vi "FPGA Sensing.vi"(8 "Error In":errorcluster, 11 "FPGA VI Reference In":refnum<k20>) -> (0 "Error Out":errorcluster, 2 "SSG Data Out":T1 {"SSG Active Current" format="%2.1f"; "PV Reactive Power (L1)" format="%2.1f"; "PV Reactive Power (L2)" format="%2.1f"; "PV Total Reactive Power" format="%2.1f"; "Gen Reactive Power (L1)" format="%2.1f"; "Gen Reactive Power (L2)" format="%2.1f"; "Gen Total Reactive Power" format="%2.1f"; "SSG Reactive Power (L1)" format="%2.1f"; "SSG Reactive Power (L2)" format="%2.1f"; "SSG Total Reactive Power" format="%2.1f"; "PV Total Current" format="%2.1f"; "PV Total Voltage" format="%2.1f"; "PV Active Power (L1)" format="%2.1f"; "PV Active Power (L2)" format="%2.1f"; "PV App Power (L1)" format="%2.1f"; "PV App Power (L2)" format="%2.1f"; "PV Total Active Power" format="%2.1f"; "PV Total App Power" format="%2.1f"; "PV Arms (L1)" format="%2.1f"; "PV Arms (L2)" format="%2.1f"; "PV Vrms (L1)" format="%2.1f"; "PV Vrms (L2)" format="%2.1f"; "Gen Total Current" format="%2.1f"; "SSG Total Current" format="%2.1f"; "Gen Total Voltage" format="%2.1f"; "SSG Total Voltage" format="%2.1f"; "Gen Active Power (L1)" format="%2.1f"; "Gen Active Power (L2)" format="%2.1f"; "SSG Active Power (L1)" format="%2.1f"; "SSG Active Power (L2)" format="%2.1f"; "Gen App Power (L1)" format="%2.1f"; "Gen App Power (L2)" format="%2.1f"; "SSG App Power (L1)" format="%2.1f"; "SSG App Power (L2)" format="%2.1f"; "Gen Total Active Power" format="%2.1f"; "Gen Total App Power" format="%2.1f"; "Gen Arms (L1)" format="%2.1f"; "Gen Arms (L2)" format="%2.1f"; "Gen Vrms (L1)" format="%2.1f"; "Gen Vrms (L2)" format="%2.1f"; "SSG Total Active Power" format="%2.1f"; "SSG Total App Power" format="%2.1f"; "SSG Arms (L1)" format="%2.1f"; "SSG Arms (L2)" format="%2.1f"; "SSG Vrms (L1)" format="%2.1f"; "SSG Vrms (L2)" format="%2.1f"})   [LabVIEW 2014]
uses:
  Controls/FPGA Data.ctl
  <vilib>/Analysis/5stat.llb/RMS (DBL).vi
  <vilib>/Utility/error.llb/Error Cluster From Error Code.vi
  <vilib>/rvi/errors/niLvFpgaAdjustHostInterfaceError.vi
  <vilib>/rvi/interface/nirviMethod/nirviMethod.xnode
  <vilib>/FPGAPlugInAG/Dynamic/niLvFpga_ReadFifo_Dynamic.vi
  <vilib>/rvi/errors/niLvFpgaMergeErrorWithErrorCode.vi
  <vilib>/Analysis/NI_AALPro.lvlib
panel:
  out "Gen Voltage":dbl[][](graph)
  out "Gen Current":dbl[][](graph)
  out "PV Voltage":dbl[][](graph)
  out "PV Current":dbl[][](graph)
  out "SSG Voltage":dbl[][](graph)
  out "SSG Current":dbl[][](graph)
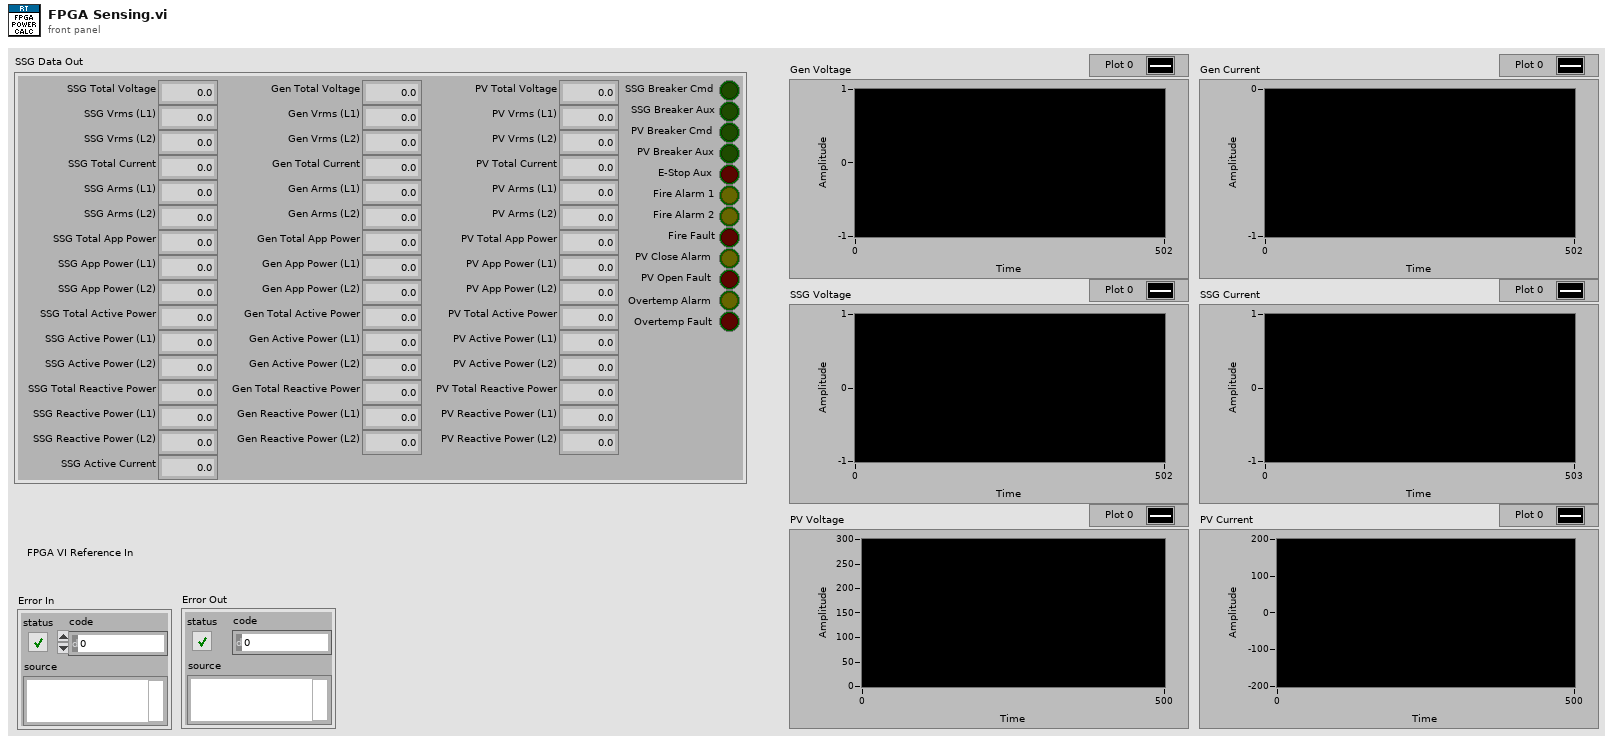
[diagram p1: front panel]
types:
  T1 = typedef "FPGA Data.ctl" = cluster{"Gen Total Voltage":dbl, "Gen Vrms (L1)":dbl, "Gen Vrms (L2)":dbl, "Gen Total Current":dbl, "Gen Arms (L1)":dbl, "Gen Arms (L2)":dbl, "Gen Total App Power":dbl, "Gen App Power (L1)":dbl, "Gen App Power (L2)":dbl, "Gen Total Active Power":dbl, "Gen Active Power (L1)":dbl, "Gen Active Power (L2)":dbl, "Gen Total Reactive Power":dbl, "Gen Reactive Power (L1)":dbl, "Gen Reactive Power (L2)":dbl, "SSG Total Voltage":dbl, "SSG Vrms (L1)":dbl, "SSG Vrms (L2)":dbl, "SSG Total Current":dbl, "SSG Arms (L1)":dbl, "SSG Arms (L2)":dbl, "SSG Total App Power":dbl, "SSG App Power (L1)":dbl, "SSG App Power (L2)":dbl, "SSG Total Active Power":dbl, "SSG Active Power (L1)":dbl, "SSG Active Power (L2)":dbl, "SSG Total Reactive Power":dbl, "SSG Reactive Power (L1)":dbl, "SSG Reactive Power (L2)":dbl, "PV Total Voltage":dbl, "PV Vrms (L1)":dbl, "PV Vrms (L2)":dbl, "PV Total Current":dbl, "PV Arms (L1)":dbl, "PV Arms (L2)":dbl, "PV Total App Power":dbl, "PV App Power (L1)":dbl, "PV App Power (L2)":dbl, "PV Total Active Power":dbl, "PV Active Power (L1)":dbl, "PV Active Power (L2)":dbl, "PV Total Reactive Power":dbl, "PV Reactive Power (L1)":dbl, "PV Reactive Power (L2)":dbl, "SSG Breaker Cmd":bool, "SSG Breaker Aux":bool, "PV Breaker Cmd":bool, "PV Breaker Aux":bool, "E-Stop Aux":bool, "Fire Alarm 1":bool, "Fire Alarm 2":bool, "Fire Fault":bool, "PV Close Alarm":bool, "SSG Active Current":dbl, "Overtemp Alarm":bool, "Overtemp Fault":bool, "PV Open Fault":bool}
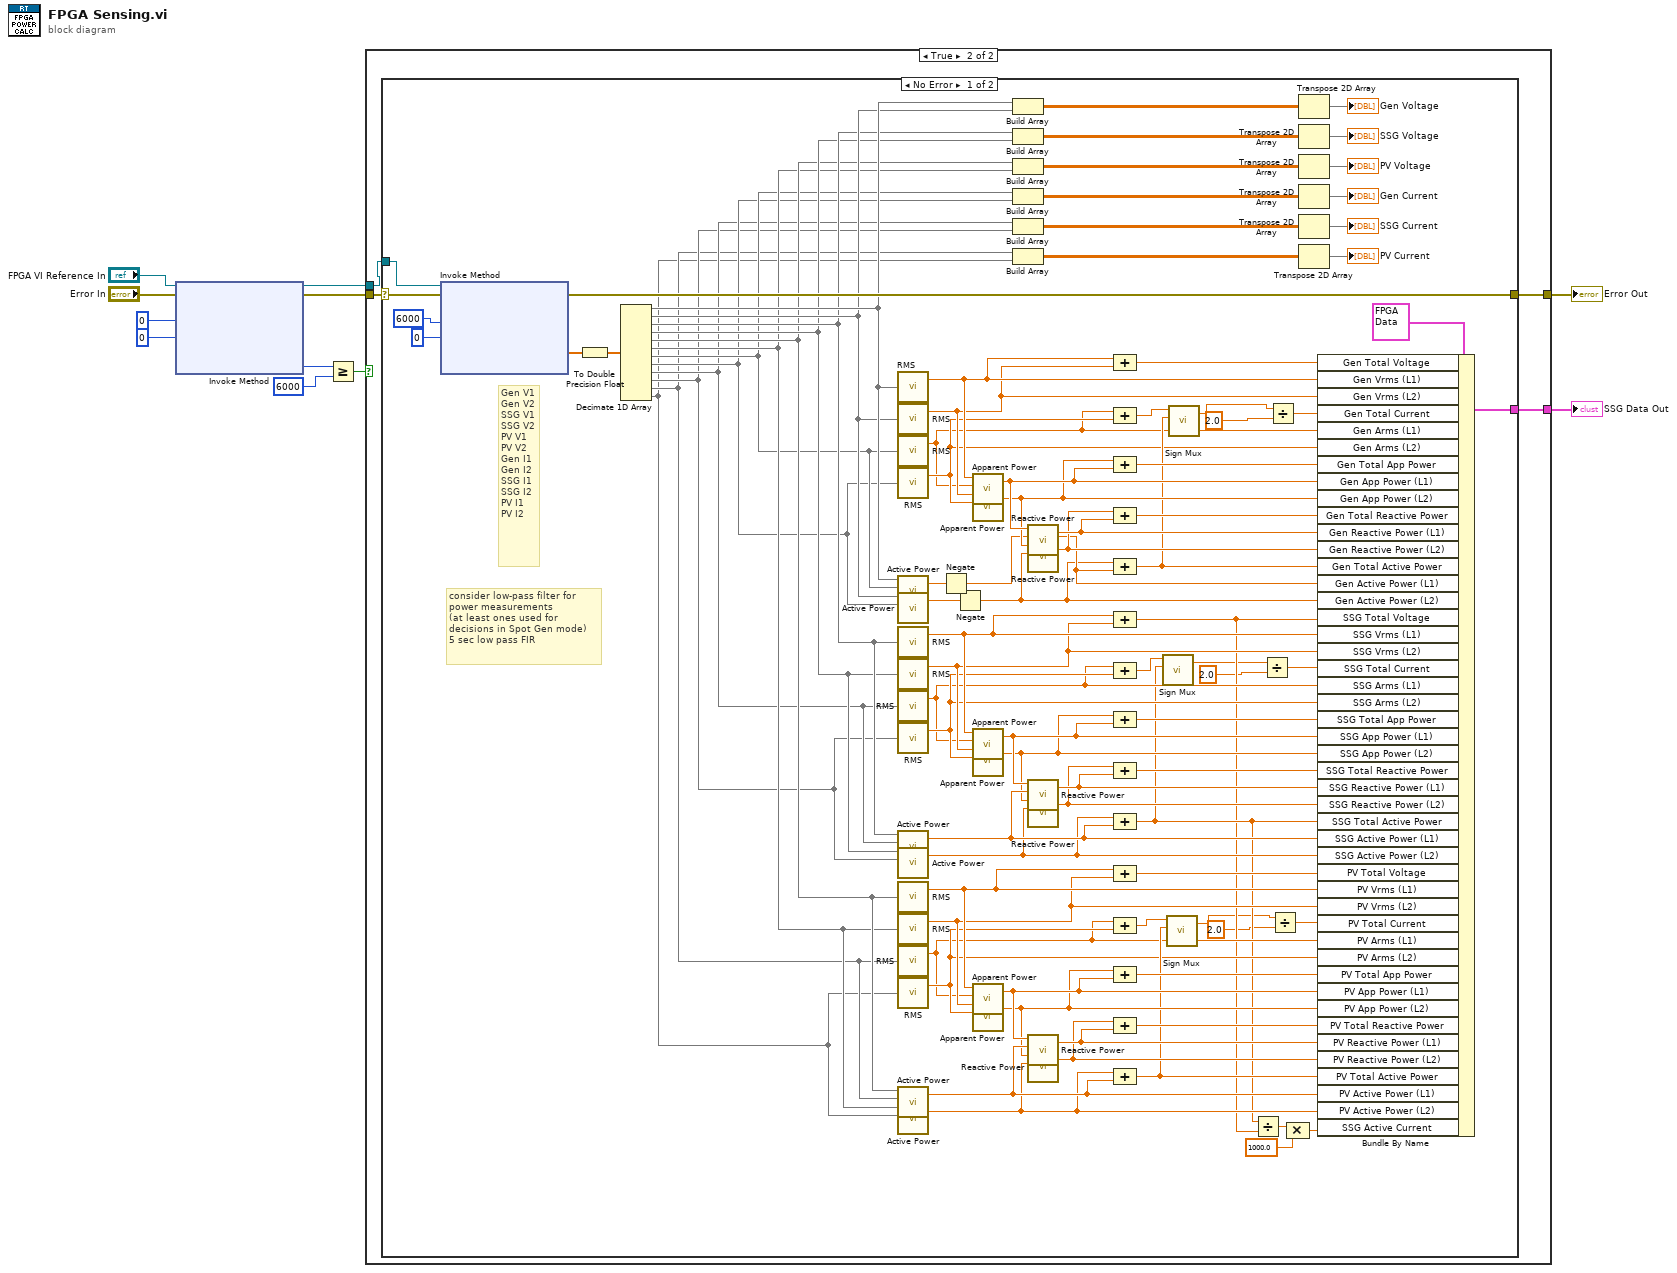
[diagram p0: block diagram]
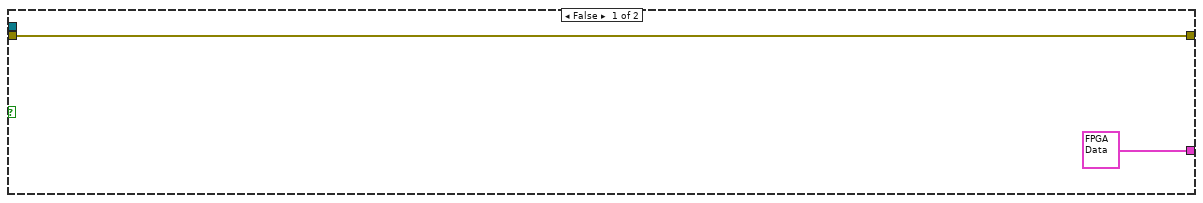
[diagram p2: hidden frame]
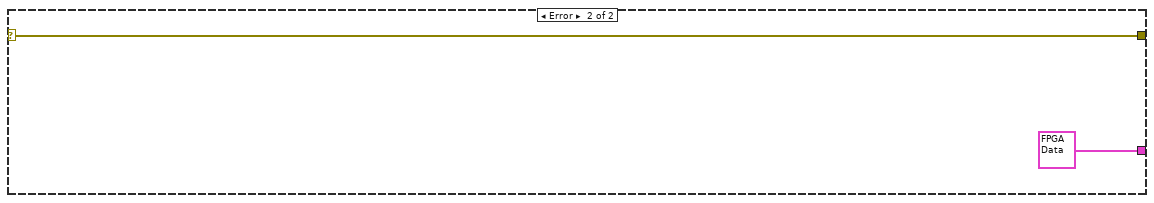
[diagram p3: hidden frame]
diagram:
  n1 = xnode "Invoke Method"("FPGA VI Reference In"="FPGA VI Reference In", "error in"="Error In", "Number of Elements"=u32 0, "Timeout (ms)"=0) -> ("FPGA VI Reference Out"=w4:refnum<k20>, "error out"=w3:errorcluster, "Elements Remaining"=w10:u32)  [unwired: 1 out]
  n2 = Greater Or Equal?(x=w10, y=u32 6000) -> (x >= y?=w5:bool)
  n3 = case shown="True" w5 {
    tunnel: w4 -> [_ w14]
    tunnel: w3 -> [w12 w17]
    tunnel: [T1 {"Gen Total Voltage"=0.0, "Gen Vrms (L1)"=0.0, "Gen Vrms (L2)"=0.0, "Gen Total Current"=0.0, "Gen Arms (L1)"=0.0, "Gen Arms (L2)"=0.0, "Gen Total App Power"=0.0, "Gen App Power (L1)"=0.0, "Gen App Power (L2)"=0.0, "Gen Total Active Power"=0.0, "Gen Active Power (L1)"=0.0, "Gen Active Power (L2)"=0.0, "Gen Total Reactive Power"=0.0, "Gen Reactive Power (L1)"=0.0, "Gen Reactive Power (L2)"=0.0, "SSG Total Voltage"=0.0, "SSG Vrms (L1)"=0.0, "SSG Vrms (L2)"=0.0, "SSG Total Current"=0.0, "SSG Arms (L1)"=0.0, "SSG Arms (L2)"=0.0, "SSG Total App Power"=0.0, "SSG App Power (L1)"=0.0, "SSG App Power (L2)"=0.0, "SSG Total Active Power"=0.0, "SSG Active Power (L1)"=0.0, "SSG Active Power (L2)"=0.0, "SSG Total Reactive Power"=0.0, "SSG Reactive Power (L1)"=0.0, "SSG Reactive Power (L2)"=0.0, "PV Total Voltage"=0.0, "PV Vrms (L1)"=0.0, "PV Vrms (L2)"=0.0, "PV Total Current"=0.0, "PV Arms (L1)"=0.0, "PV Arms (L2)"=0.0, "PV Total App Power"=0.0, "PV App Power (L1)"=0.0, "PV App Power (L2)"=0.0, "PV Total Active Power"=0.0, "PV Active Power (L1)"=0.0, "PV Active Power (L2)"=0.0, "PV Total Reactive Power"=0.0, "PV Reactive Power (L1)"=0.0, "PV Reactive Power (L2)"=0.0, "SSG Breaker Cmd"=FALSE, "SSG Breaker Aux"=FALSE, "PV Breaker Cmd"=FALSE, "PV Breaker Aux"=FALSE, "E-Stop Aux"=FALSE, "Fire Alarm 1"=FALSE, "Fire Alarm 2"=FALSE, "Fire Fault"=FALSE, "PV Close Alarm"=FALSE, "SSG Active Current"=0.0, "Overtemp Alarm"=FALSE, "Overtemp Fault"=FALSE, "PV Open Fault"=FALSE} ("SSG Data Out") w16] -> w2
    tunnel: [w12 w15] -> w1
    frame False {
    }
    frame True {
      n4 = case shown="No Error" w17 {
        selector: w17 -> [w106 w110]
        tunnel: [w107 T1 {"Gen Total Voltage"=0.0, "Gen Vrms (L1)"=0.0, "Gen Vrms (L2)"=0.0, "Gen Total Current"=0.0, "Gen Arms (L1)"=0.0, "Gen Arms (L2)"=0.0, "Gen Total App Power"=0.0, "Gen App Power (L1)"=0.0, "Gen App Power (L2)"=0.0, "Gen Total Active Power"=0.0, "Gen Active Power (L1)"=0.0, "Gen Active Power (L2)"=0.0, "Gen Total Reactive Power"=0.0, "Gen Reactive Power (L1)"=0.0, "Gen Reactive Power (L2)"=0.0, "SSG Total Voltage"=0.0, "SSG Vrms (L1)"=0.0, "SSG Vrms (L2)"=0.0, "SSG Total Current"=0.0, "SSG Arms (L1)"=0.0, "SSG Arms (L2)"=0.0, "SSG Total App Power"=0.0, "SSG App Power (L1)"=0.0, "SSG App Power (L2)"=0.0, "SSG Total Active Power"=0.0, "SSG Active Power (L1)"=0.0, "SSG Active Power (L2)"=0.0, "SSG Total Reactive Power"=0.0, "SSG Reactive Power (L1)"=0.0, "SSG Reactive Power (L2)"=0.0, "PV Total Voltage"=0.0, "PV Vrms (L1)"=0.0, "PV Vrms (L2)"=0.0, "PV Total Current"=0.0, "PV Arms (L1)"=0.0, "PV Arms (L2)"=0.0, "PV Total App Power"=0.0, "PV App Power (L1)"=0.0, "PV App Power (L2)"=0.0, "PV Total Active Power"=0.0, "PV Active Power (L1)"=0.0, "PV Active Power (L2)"=0.0, "PV Total Reactive Power"=0.0, "PV Reactive Power (L1)"=0.0, "PV Reactive Power (L2)"=0.0, "SSG Breaker Cmd"=FALSE, "SSG Breaker Aux"=FALSE, "PV Breaker Cmd"=FALSE, "PV Breaker Aux"=FALSE, "E-Stop Aux"=FALSE, "Fire Alarm 1"=FALSE, "Fire Alarm 2"=FALSE, "Fire Fault"=FALSE, "PV Close Alarm"=FALSE, "SSG Active Current"=0.0, "Overtemp Alarm"=FALSE, "Overtemp Fault"=FALSE, "PV Open Fault"=FALSE} ("SSG Data Out")] -> w16
        tunnel: [w109 w110] -> w15
        tunnel: w14 -> [w18 _]
        frame No Error {
          # "consider low-pass filter for \npower measurements\n(at least ones used for \ndecisions in Spot Gen mode)\n5 sec low pass FIR"
          # "Gen V1\nGen V2\nSSG V1\nSSG V2\nPV V1\nPV V2\nGen I1\nGen I2\nSSG I1\nSSG I2\nPV I1\nPV I2"
          n5 = xnode "Invoke Method"("FPGA VI Reference In"=w18, "error in"=w106, "Number of Elements"=u32 6000, "Timeout (ms)"=0) -> ("error out"=w109:errorcluster, "Data"=w103:sgl[])  [unwired: 2 out]
          n6 = To Double Precision Float(number=w103) -> (double precision float=w102:dbl[])
          n7 = Decimate 1D Array(w102) -> (w101:dbl[], w100:dbl[], w99:dbl[], w98:dbl[], w97:dbl[], w96:dbl[], w95:dbl[], w94:dbl[], w93:dbl[], w92:dbl[], w91:dbl[], w90:dbl[])
          n8 = call-poly <vilib>:"RMS.vi"("X"=w101) -> ("rms value"=w46:dbl)  [unwired: 1 out]
          n9 = call-poly <vilib>:"RMS.vi"("X"=w100) -> ("rms value"=w45:dbl)  [unwired: 1 out]
          n10 = call-poly <vilib>:"RMS.vi"("X"=w95) -> ("rms value"=w35:dbl)  [unwired: 1 out]
          n11 = call-poly <vilib>:"RMS.vi"("X"=w94) -> ("rms value"=w43:dbl)  [unwired: 1 out]
          n12 = call "Active Power.vi"("Current Waveform"=w95, "Voltage Waveform"=w101) -> ("Active Power"=w73:dbl)  [unwired: 3 in]
          n13 = call "Active Power.vi"("Current Waveform"=w94, "Voltage Waveform"=w100) -> ("Active Power"=w72:dbl)  [unwired: 3 in]
          n14 = call-poly <vilib>:"RMS.vi"("X"=w99) -> ("rms value"=w48:dbl)  [unwired: 1 out]
          n15 = call-poly <vilib>:"RMS.vi"("X"=w98) -> ("rms value"=w47:dbl)  [unwired: 1 out]
          n16 = call-poly <vilib>:"RMS.vi"("X"=w93) -> ("rms value"=w37:dbl)  [unwired: 1 out]
          n17 = call-poly <vilib>:"RMS.vi"("X"=w92) -> ("rms value"=w41:dbl)  [unwired: 1 out]
          n18 = call "Active Power.vi"("Current Waveform"=w93, "Voltage Waveform"=w99) -> ("Active Power"=w66:dbl)  [unwired: 3 in]
          n19 = call "Active Power.vi"("Current Waveform"=w92, "Voltage Waveform"=w98) -> ("Active Power"=w64:dbl)  [unwired: 3 in]
          n20 = call-poly <vilib>:"RMS.vi"("X"=w97) -> ("rms value"=w51:dbl)  [unwired: 1 out]
          n21 = call-poly <vilib>:"RMS.vi"("X"=w96) -> ("rms value"=w50:dbl)  [unwired: 1 out]
          n22 = call-poly <vilib>:"RMS.vi"("X"=w91) -> ("rms value"=w36:dbl)  [unwired: 1 out]
          n23 = call-poly <vilib>:"RMS.vi"("X"=w90) -> ("rms value"=w39:dbl)  [unwired: 1 out]
          n24 = call "Active Power.vi"("Current Waveform"=w91, "Voltage Waveform"=w97) -> ("Active Power"=w58:dbl)  [unwired: 3 in]
          n25 = call "Active Power.vi"("Current Waveform"=w90, "Voltage Waveform"=w96) -> ("Active Power"=w56:dbl)  [unwired: 3 in]
          n26 = Negate(x=w73) -> (-x=w34:dbl)
          n27 = Negate(x=w72) -> (-x=w33:dbl)
          n28 = call "Apparent Power.vi"("Arms"=w35, "Vrms"=w46) -> ("Apparent Power"=w74:dbl)  [unwired: 3 in]
          n29 = call "Apparent Power.vi"("Arms"=w43, "Vrms"=w45) -> ("Apparent Power"=w71:dbl)  [unwired: 3 in]
          n30 = call "Apparent Power.vi"("Arms"=w37, "Vrms"=w48) -> ("Apparent Power"=w67:dbl)  [unwired: 3 in]
          n31 = call "Apparent Power.vi"("Arms"=w41, "Vrms"=w47) -> ("Apparent Power"=w65:dbl)  [unwired: 3 in]
          n32 = call "Apparent Power.vi"("Arms"=w36, "Vrms"=w51) -> ("Apparent Power"=w59:dbl)  [unwired: 3 in]
          n33 = call "Apparent Power.vi"("Arms"=w39, "Vrms"=w50) -> ("Apparent Power"=w57:dbl)  [unwired: 3 in]
          n34 = Build Array(w101, w100) -> (w89:dbl[][])
          n35 = Build Array(w99, w98) -> (w88:dbl[][])
          n36 = Build Array(w97, w96) -> (w87:dbl[][])
          n37 = Build Array(w95, w94) -> (w86:dbl[][])
          n38 = Build Array(w93, w92) -> (w85:dbl[][])
          n39 = Build Array(w91, w90) -> (w84:dbl[][])
          n40 = call "Reactive Power.vi"("Active Power"=w34, "Apparent Power"=w74) -> ("Reactive Power"=w69:dbl)  [unwired: 3 in]
          n41 = call "Reactive Power.vi"("Active Power"=w33, "Apparent Power"=w71) -> ("Reactive Power"=w68:dbl)  [unwired: 3 in]
          n42 = call "Reactive Power.vi"("Active Power"=w66, "Apparent Power"=w67) -> ("Reactive Power"=w62:dbl)  [unwired: 3 in]
          n43 = call "Reactive Power.vi"("Active Power"=w64, "Apparent Power"=w65) -> ("Reactive Power"=w61:dbl)  [unwired: 3 in]
          n44 = call "Reactive Power.vi"("Active Power"=w58, "Apparent Power"=w59) -> ("Reactive Power"=w55:dbl)  [unwired: 3 in]
          n45 = call "Reactive Power.vi"("Active Power"=w56, "Apparent Power"=w57) -> ("Reactive Power"=w54:dbl)  [unwired: 3 in]
          n46 = Compound Arithmetic op=ADD(w46, w45) -> (w44:dbl)
          n47 = Compound Arithmetic op=ADD(w35, w43) -> (w42:dbl)
          n48 = Compound Arithmetic op=ADD(w71, w74) -> (w77:dbl)
          n49 = Compound Arithmetic op=ADD(w68, w69) -> (w70:dbl)
          n50 = Compound Arithmetic op=ADD(w33, w34) -> (w53:dbl)
          n51 = Compound Arithmetic op=ADD(w48, w47) -> (w31:dbl)
          n52 = Compound Arithmetic op=ADD(w37, w41) -> (w40:dbl)
          n53 = Compound Arithmetic op=ADD(w65, w67) -> (w76:dbl)
          n54 = Compound Arithmetic op=ADD(w61, w62) -> (w63:dbl)
          n55 = Compound Arithmetic op=ADD(w64, w66) -> (w32:dbl)
          n56 = Compound Arithmetic op=ADD(w51, w50) -> (w49:dbl)
          n57 = Compound Arithmetic op=ADD(w36, w39) -> (w38:dbl)
          n58 = Compound Arithmetic op=ADD(w57, w59) -> (w75:dbl)
          n59 = Compound Arithmetic op=ADD(w54, w55) -> (w60:dbl)
          n60 = Compound Arithmetic op=ADD(w56, w58) -> (w52:dbl)
          n61 = call "Sign Mux.vi"("Signed Number B"=w32, "Unsigned Number A"=w40) -> ("Signed Number A"=w26:dbl)  [unwired: 3 in]
          n62 = call "Sign Mux.vi"("Signed Number B"=w52, "Unsigned Number A"=w38) -> ("Signed Number A"=w22:dbl)  [unwired: 3 in]
          n63 = call "Sign Mux.vi"("Signed Number B"=w53, "Unsigned Number A"=w42) -> ("Signed Number A"=w20:dbl)  [unwired: 3 in]
          n64 = Divide(x=w32, y=w31) -> (x/y=w30:dbl)
          n65 = Divide(x=w26, y=2.0) -> (x/y=w27:dbl)
          n66 = Divide(x=w20, y=2.0) -> (x/y=w19:dbl)
          n67 = Divide(x=w22, y=2.0) -> (x/y=w21:dbl)
          n68 = Compound Arithmetic op=MULTIPLY(w30, 1000.0 ("value")) -> (w29:dbl)
          n69 = Transpose 2D Array(2D array=w89) -> (transposed array=→"Gen Voltage":dbl[][])
          n70 = Transpose 2D Array(2D array=w88) -> (transposed array=→"SSG Voltage":dbl[][])
          n71 = Transpose 2D Array(2D array=w87) -> (transposed array=→"PV Voltage":dbl[][])
          n72 = Transpose 2D Array(2D array=w86) -> (transposed array=→"Gen Current":dbl[][])
          n73 = Transpose 2D Array(2D array=w85) -> (transposed array=→"SSG Current":dbl[][])
          n74 = Transpose 2D Array(2D array=w84) -> (transposed array=→"PV Current":dbl[][])
          n75 = Bundle By Name(cluster=T1 {"Gen Total Voltage"=0.0, "Gen Vrms (L1)"=0.0, "Gen Vrms (L2)"=0.0, "Gen Total Current"=0.0, "Gen Arms (L1)"=0.0, "Gen Arms (L2)"=0.0, "Gen Total App Power"=0.0, "Gen App Power (L1)"=0.0, "Gen App Power (L2)"=0.0, "Gen Total Active Power"=0.0, "Gen Active Power (L1)"=0.0, "Gen Active Power (L2)"=0.0, "Gen Total Reactive Power"=0.0, "Gen Reactive Power (L1)"=0.0, "Gen Reactive Power (L2)"=0.0, "SSG Total Voltage"=0.0, "SSG Vrms (L1)"=0.0, "SSG Vrms (L2)"=0.0, "SSG Total Current"=0.0, "SSG Arms (L1)"=0.0, "SSG Arms (L2)"=0.0, "SSG Total App Power"=0.0, "SSG App Power (L1)"=0.0, "SSG App Power (L2)"=0.0, "SSG Total Active Power"=0.0, "SSG Active Power (L1)"=0.0, "SSG Active Power (L2)"=0.0, "SSG Total Reactive Power"=0.0, "SSG Reactive Power (L1)"=0.0, "SSG Reactive Power (L2)"=0.0, "PV Total Voltage"=0.0, "PV Vrms (L1)"=0.0, "PV Vrms (L2)"=0.0, "PV Total Current"=0.0, "PV Arms (L1)"=0.0, "PV Arms (L2)"=0.0, "PV Total App Power"=0.0, "PV App Power (L1)"=0.0, "PV App Power (L2)"=0.0, "PV Total Active Power"=0.0, "PV Active Power (L1)"=0.0, "PV Active Power (L2)"=0.0, "PV Total Reactive Power"=0.0, "PV Reactive Power (L1)"=0.0, "PV Reactive Power (L2)"=0.0, "SSG Breaker Cmd"=FALSE, "SSG Breaker Aux"=FALSE, "PV Breaker Cmd"=FALSE, "PV Breaker Aux"=FALSE, "E-Stop Aux"=FALSE, "Fire Alarm 1"=FALSE, "Fire Alarm 2"=FALSE, "Fire Fault"=FALSE, "PV Close Alarm"=FALSE, "SSG Active Current"=0.0, "Overtemp Alarm"=FALSE, "Overtemp Fault"=FALSE, "PV Open Fault"=FALSE} ("SSG Data Out"), "Gen Total Voltage"=w44, "Gen Vrms (L1)"=w46, "Gen Vrms (L2)"=w45, "Gen Total Current"=w19, "Gen Arms (L1)"=w35, "Gen Arms (L2)"=w43, "Gen Total App Power"=w77, "Gen App Power (L1)"=w74, "Gen App Power (L2)"=w71, "Gen Total Reactive Power"=w70, "Gen Reactive Power (L1)"=w69, "Gen Reactive Power (L2)"=w68, "Gen Total Active Power"=w53, "Gen Active Power (L1)"=w34, "Gen Active Power (L2)"=w33, "SSG Total Voltage"=w31, "SSG Vrms (L1)"=w48, "SSG Vrms (L2)"=w47, "SSG Total Current"=w27, "SSG Arms (L1)"=w37, "SSG Arms (L2)"=w41, "SSG Total App Power"=w76, "SSG App Power (L1)"=w67, "SSG App Power (L2)"=w65, "SSG Total Reactive Power"=w63, "SSG Reactive Power (L1)"=w62, "SSG Reactive Power (L2)"=w61, "SSG Total Active Power"=w32, "SSG Active Power (L1)"=w66, "SSG Active Power (L2)"=w64, "PV Total Voltage"=w49, "PV Vrms (L1)"=w51, "PV Vrms (L2)"=w50, "PV Total Current"=w21, "PV Arms (L1)"=w36, "PV Arms (L2)"=w39, "PV Total App Power"=w75, "PV App Power (L1)"=w59, "PV App Power (L2)"=w57, "PV Total Reactive Power"=w60, "PV Reactive Power (L1)"=w55, "PV Reactive Power (L2)"=w54, "PV Total Active Power"=w52, "PV Active Power (L1)"=w58, "PV Active Power (L2)"=w56, "SSG Active Current"=w29) -> (w107:T1)
        }
        frame Error {
        }
      }
    }
  }
  "SSG Data Out" <- w2
  "Error Out" <- w1
